vi "prepareUpload.vi"(10 "progOnly":bool, 11 "loopData":T1) -> (3 "code":u8[][](array[numeric]))   [LabVIEW 2014]
uses:
  typeDefs/loopDataType.ctl
  typeDefs/editControl.ctl
  typeDefs/variantFlat.ctl
  typeDefs/pictChooser.ctl
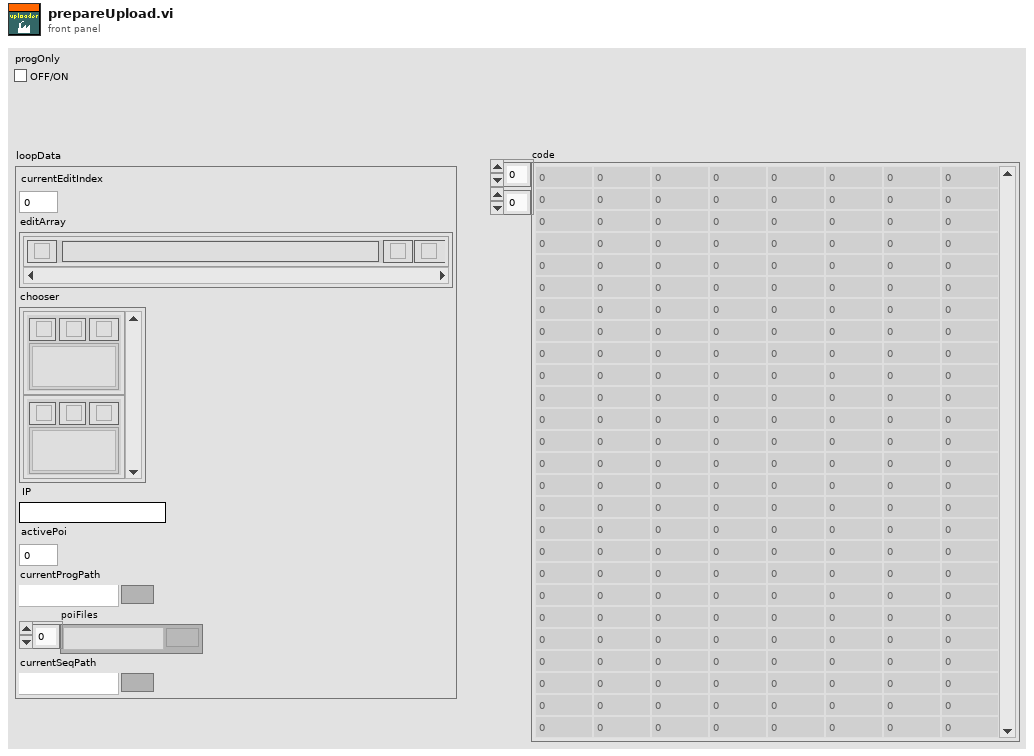
[diagram p1: front panel]
types:
  T1 = typedef "loopDataType.ctl" = cluster{"currentEditIndex":i32, "editArray":T2[], "chooser":T4[], "IP":string, "activePoi":i32, "currentProgPath":path, "poiFiles":path[], "currentSeqPath":path}
  T2 = typedef "editControl.ctl" = cluster{"edit":bool, "info":string, "variantFlat":T3, "codeCluster":cluster{"code":u8[][]}, "del":bool, "ins":bool}
  T3 = typedef "variantFlat.ctl" = cluster{"type string":i16[], "data string":string}
  T4 = typedef "pictChooser.ctl" = cluster{"2D Picture":picture, "load":bool, "Path":path, "Bitmap":u32[][], "del":bool, "paint":bool}
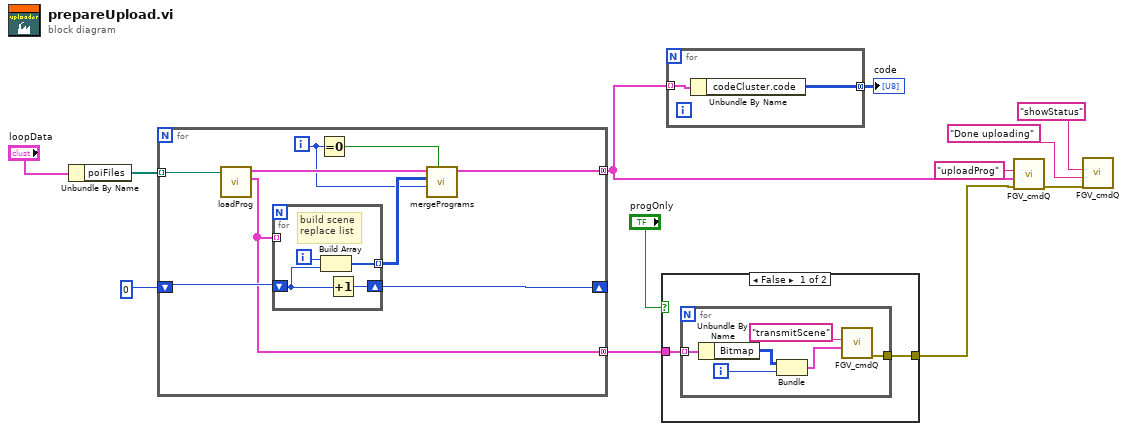
[diagram p0: block diagram]
diagram:
  n1 = Unbundle By Name("loopData") -> ("poiFiles"=w11:path[])
  n2 = for {
    tunnel: w11 -> [w21] mode=indexing
    shift-right: [w18] -> _
    shift-left: 0 -> [w17]
    tunnel: [w15] -> w8 mode=concatenating
    tunnel: [w14] -> w6 mode=concatenating
    i -> [w13]
    n3 = call "loadProg.vi"("selected path"=w21) -> ("scenes"=w15:T4[], "editArray"=w20:T2[])  [unwired: 8 in, 1 out]
    n4 = for {
      tunnel: w15 -> [_] mode=indexing
      shift-right: [w24] -> w18
      shift-left: w17 -> [w23]
      tunnel: [w22] -> w16 mode=indexing
      i -> [w25]
      # "build scene\nreplace list"
      n5 = Build Array(w25, w23) -> (w22:i32[])
      n6 = Increment(x=w23) -> (x+1=w24:i32)
    }
    n7 = Equal To 0?(x=w13) -> (x = 0?=w19:bool)
    n8 = call "mergePrograms.vi"("init"=w19, "syncLabel"=w13, "sceneReplaceList"=w16, "editArray"=w20) -> ("editRecalc"=w14:T2[])  [unwired: 7 in]
  }
  n9 = case shown="False" "progOnly" {
    tunnel: w8 -> [w27 _]
    tunnel: [w26 _] -> w4
    frame False {
      n10 = for {
        tunnel: w27 -> [w31] mode=indexing
        tunnel: [w28] -> w26
        i -> [w30]
        n11 = Unbundle By Name(w31) -> ("Bitmap"=w29:u32[][])
        n12 = Bundle("Bitmap"=w29, w30) -> (w32:cluster{"Bitmap":u32[][], i32})  [unwired: 1 in]
        n13 = call "FGV_cmdQ.vi"("dataIn"=w32, "actionIn"="transmitScene") -> ("error out"=w28:errorcluster)  [unwired: 8 in, 1 out]
      }
    }
    frame True {
    }
  }
  n14 = for {
    tunnel: w6 -> [w35] mode=indexing
    tunnel: [w34] -> w5 mode=concatenating
    n15 = Unbundle By Name(w35) -> ("codeCluster.code"=w34:u8[][])
  }
  "code" <- w5
  n16 = call "FGV_cmdQ.vi"("error in (no error)"=w4, "dataIn"=w6, "actionIn"="uploadProg") -> ("error out"=w3:errorcluster)  [unwired: 7 in, 1 out]
  n17 = call "FGV_cmdQ.vi"("error in (no error)"=w3, "dataIn"="Done uploading" ("actionIn"), "actionIn"="showStatus") -> ()  [unwired: 7 in, 2 out]
